vi "Update Distance with Step.vi"(8 "error in (no error)":errorcluster, 10 "Step":i32, 11 "Picture Ring in":refnum<class "Node.lvclass">) -> (0 "error out":errorcluster, 2 "Type":T1, 3 "Picture Ring out":refnum<class "Node.lvclass">)   [LabVIEW 2019, in "Node.lvclass"]
uses:
  Node.lvclass
  Shared/Node Type--enum.ctl
  Node.lvclass/Node.ctl
  Shared/Shared.lvlib
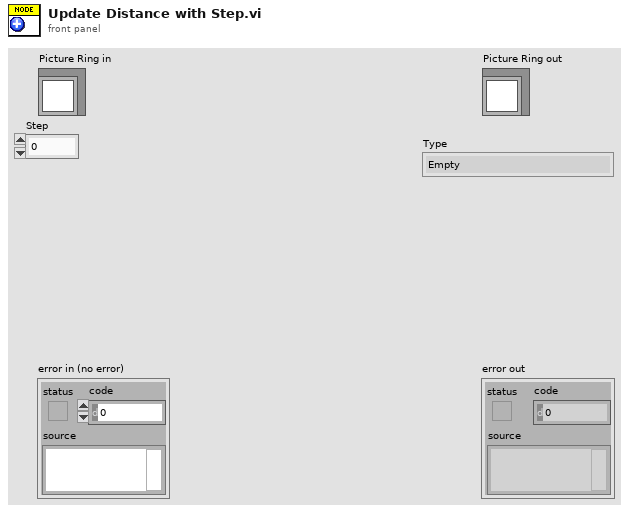
[diagram p1: front panel]
types:
  T1 = typedef "Shared.lvlib/Node Type--enum.ctl" = enum16{"Empty", "Blocked", "Start", "End", "Path"}
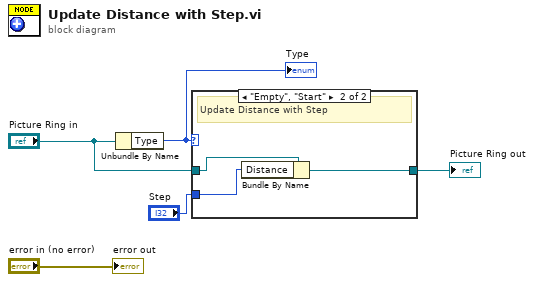
[diagram p0: block diagram]
diagram:
  n1 = Unbundle By Name("Picture Ring in") -> ("Type"=w5:T1)
  "Type" <- w5
  n2 = case shown="\"Empty\", \"Start\"" w5 {
    tunnel: [w6 w8] -> w4
    tunnel: "Picture Ring in" -> [w6 w9]
    tunnel: "Step" -> [_ w7]
    frame "Blocked", "End", Default {
      # "No Operation"
    }
    frame "Empty", "Start" {
      # "Update Distance with Step"
      n3 = Bundle By Name(cluster=w9, "Distance"=w7) -> (w8:refnum<class "Node.lvclass">)
    }
  }
  "Picture Ring out" <- w4
  "error out" <- "error in (no error)"
